vi "Pre Launch Init.vi"(11 "Simple Chat in":refnum<class "Simple Chat.lvclass">) -> (0 "error out":errorcluster, 3 "Simple Chat out":refnum<class "Simple Chat.lvclass">)   [LabVIEW 2020, in "Simple Chat.lvlib" / "Simple Chat.lvclass"]
doc: "(<B>Filename</B>: Actor Framework.lvlib:Actor.lvclass:Pre Launch Init.vi)\n\nDefines behavior that occurs after the Launch Nested Actor method is invoked but before the actor's Actor Core method begins running.\n\nBy default, this method does nothing. A descendant class may override it to define behavior."
uses:
  Simple Chat.lvclass
  C:/Program Files/National Instruments/LabVIEW 2020/vi.lib/ActorFramework/Actor/Actor.lvclass
  Actor Pub Sub Channels/Pub Sub Status Message/Pub Sub Status Message.lvclass
  Chat Messages Interface/Chat Messages Interface.lvclass
  <vilib>/ActorFramework/Stop Msg/Stop Msg.lvclass
  Message Reciever Interface/Message Receiver Interface.lvclass
  <vilib>/ActorFramework/Actor/Actor.lvclass/Actor.ctl
  <vilib>/ActorFramework/Message Enqueuer/Message Enqueuer.lvclass/Message Enqueuer.ctl
  Simple Chat.lvclass/Simple Chat.ctl
  848bf2ce-151b-44f6-88e3-c0d6abaf681b.vi
  bd6d6e65-3883-49ee-af7e-76626c1ce84d.vi
  <vilib>/ActorFramework/Message Enqueuer/Init from Existing Queue.vi
  bd6d6e65-3883-49ee-af7e-76626c1ce84d.vi/ab9dd782-548d-4861-b01d-d668ac712bc7.vi
  Actor Pub Sub Channels/Helpers/Subscribe Actor to Class Topic.vi
  Actor Pub Sub Channels/Helpers/Subscribe Actor to Topic.vi
  <vilib>/ActorFramework/Actor/Actor.lvclass
  <vilib>/ActorFramework/Message Enqueuer/Message Enqueuer.lvclass
  Actor Pub Sub Channels/Actor Pub Sub Channels.lvlib
  Actor Pub Sub Channels/Pub Sub Message Channel/Pub Sub Message Channel.lvclass
  C:/Program Files/National Instruments/LabVIEW 2020/vi.lib/ActorFramework/Message/Message.lvclass
  C:/Program Files/National Instruments/LabVIEW 2020/vi.lib/ActorFramework/Stop Msg/Stop Msg.lvclass
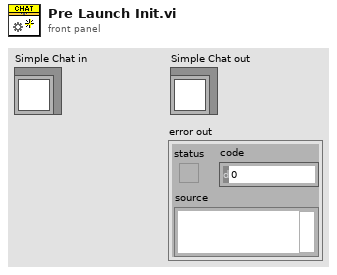
[diagram p1: front panel]
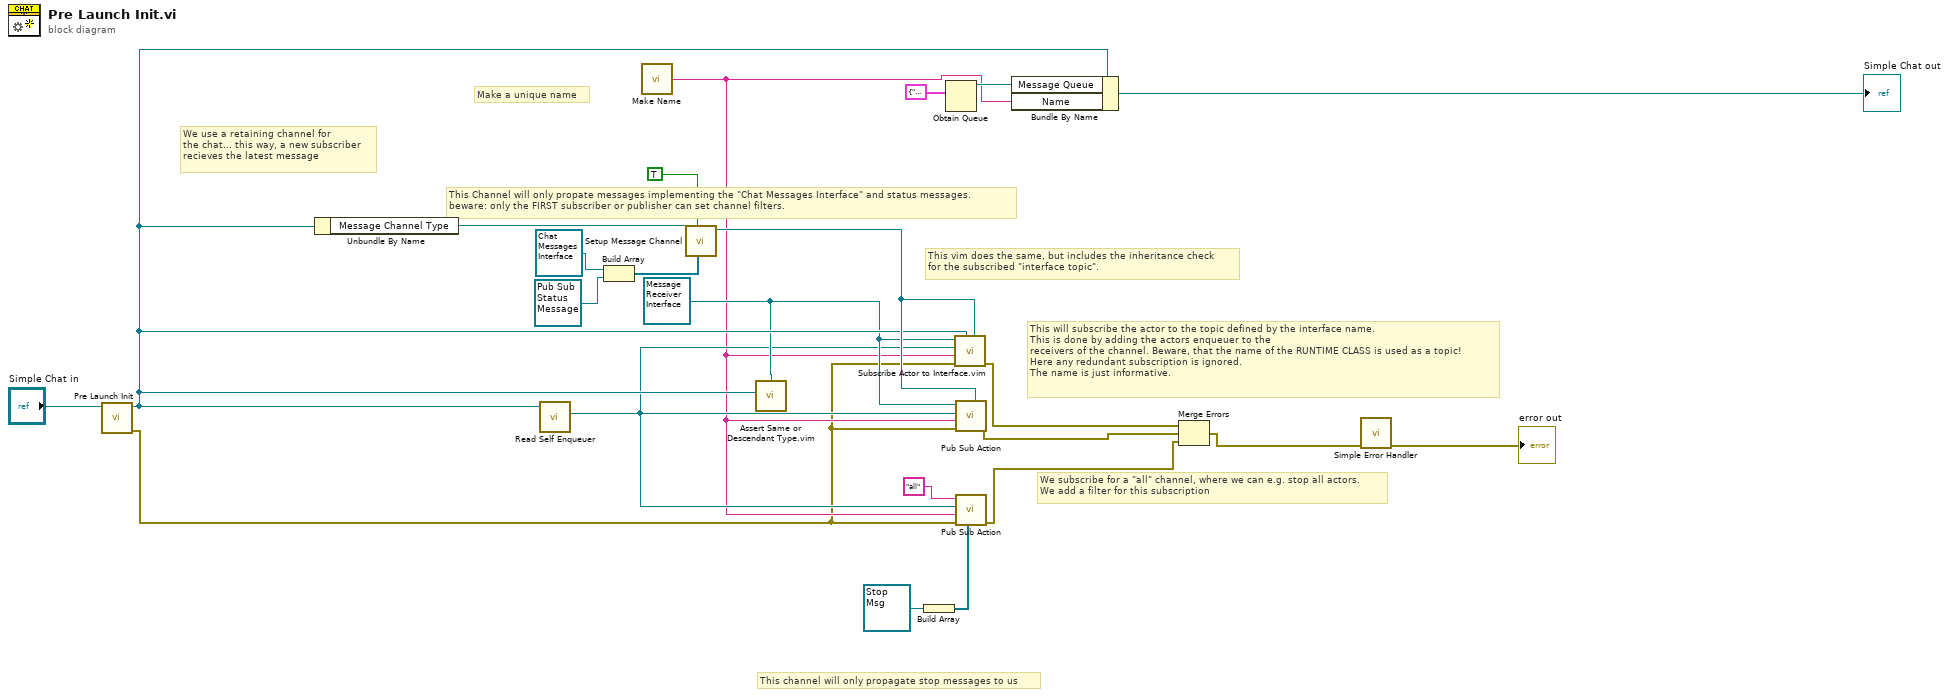
[diagram p0: block diagram]
diagram:
  w11 = refnum<class "Message Receiver Interface.lvclass"> refnum ("Simple Chat.lvlib:Message Reciever Interface.lvclass")
  # "This Channel will only propate messages implementing the \"Chat Messages Interface\" and status messages.\nbeware: only the FIRST subscriber or publisher can set channel filters."
  # "This channel will only propagate stop messages to us"
  # "Make a unique name"
  # "We subscribe for a \"all\" channel, where we can e.g. stop all actors.\nWe add a filter for this subscription"
  # "We use a retaining channel for\nthe chat... this way, a new subscriber\nrecieves the latest message"
  # "This vim does the same, but includes the inheritance check\nfor the subscribed \"interface topic\"."
  # "This will subscribe the actor to the topic defined by the interface name.\nThis is done by adding the actors enqueuer to the\nreceivers of the channel. Beware, that the name of the RUNTIME CLASS is used as a topic!\nHere any redundant subscription is ignored.\nThe name is just informative."
  n1 = call-parent "Pre Launch Init.vi"("Actor in"="Simple Chat in") -> ("error out"=w8:errorcluster, "Actor out"=w12:refnum<class "Simple Chat.lvclass">)  [unwired: 9 in]
  n2 = Unbundle By Name(w12) -> ("Message Channel Type"=w16:refnum<class "Pub Sub Message Channel.lvclass">)
  n3 = call <vilib>:"Read Self Enqueuer.vi"("Actor"=w12) -> ("Self Enqueuer"=w10:refnum<class "Message Enqueuer.lvclass">)  [unwired: 10 in]
  n4 = Build Array(refnum<class "Chat Messages Interface.lvclass"> refnum ("Simple Chat.lvlib:Chat Messages Interface.lvclass"), refnum<class "Pub Sub Status Message.lvclass"> refnum ("Actor Pub Sub Channels.lvlib:Pub Sub Status Message.lvclass")) -> (w2:refnum<class>[])
  n5 = call "Make Name.vi"() -> ("Actor Name"=w9:string)
  n6 = call "Setup Message Channel.vi"("Included (All)"=w2, "Emit Status Messages (F)"=TRUE ("Emit Status Messages"), "Pub Sub Message Channel in"=w16) -> ("Pub Sub Message Channel out"=w13:refnum<class "Pub Sub Message Channel.lvclass">)  [unwired: 7 in, 1 out]
  n7 = call "Assert Same or Descendant Type.vim"("ancestor type"=w11, "value in"=w12) -> ()  [unwired: 7 in, 1 out]
  n8 = Build Array(refnum<class "Stop Msg.lvclass"> refnum ("Actor Framework:Stop Msg")) -> (w17:refnum<class "Stop Msg.lvclass">[])
  n9 = Obtain Queue(element data type=cluster{"Sender":string, "Message":string} {"Sender"="", "Message"=""}) -> (queue out=w20:refnum<queue>)  [unwired: 4 in, 2 out]
  n10 = call "Subscribe Actor to Interface.vim"("Channel Class"=w13, "Actor"=w12, "error in (no error)"=w8, "Name"=w9, "Receivers Enqueuer"=w10, "Topic"=w11) -> ("error out"=w15:errorcluster)  [unwired: 4 in, 1 out]
  n11 = call-poly "Pub Sub Action.vi"("Channel Class"=w13, "error in (no error)"=w8, "Name"=w9, "Receivers Enqueuer"=w10, "Topic"=w11) -> ("error out"=w14:errorcluster)  [unwired: 5 in, 1 out]
  n12 = call-poly "Pub Sub Action.vi"("Included (All)"=w17, "error in (no error)"=w8, "Name"=w9, "Receivers Enqueuer"=w10, "Topic"="all") -> ("error out"=w6:errorcluster)  [unwired: 4 in, 2 out]
  n13 = Bundle By Name(cluster=w12, "Message Queue"=w20, "Name"=w9) -> (→"Simple Chat out":refnum<class "Simple Chat.lvclass">)
  n14 = Merge Errors(w15, w14, w6) -> (w7:errorcluster)
  n15 = call <vilib>:"Simple Error Handler.vi"("error in (no error)"=w7) -> ("error out"=→"error out":errorcluster)  [unwired: 4 in, 4 out]
